vi "Close.vi"(8 "error in (no error)":errorcluster, 11 "Motions in":refnum<class "Motions.lvclass">) -> (0 "error out":errorcluster, 3 "Motions out":refnum<class "Motions.lvclass">)   [LabVIEW 2016, in "Hardware.lvlib" / "Motions.lvlib" / "Motions.lvclass"]
uses:
  <userlib>/Common Components/Hardware/Abstract System/Motions/Motions/Motions.lvclass
  <userlib>/Common Components/Hardware/Abstract System/Motions/Motions/Motions.lvclass/Motions.ctl
  <userlib>/Common Components/Hardware/Motor/Motor/Motor.lvclass
  <userlib>/Common Components/TriggerAction Q/TriggerAction Q/TriggerAction Q.lvclass
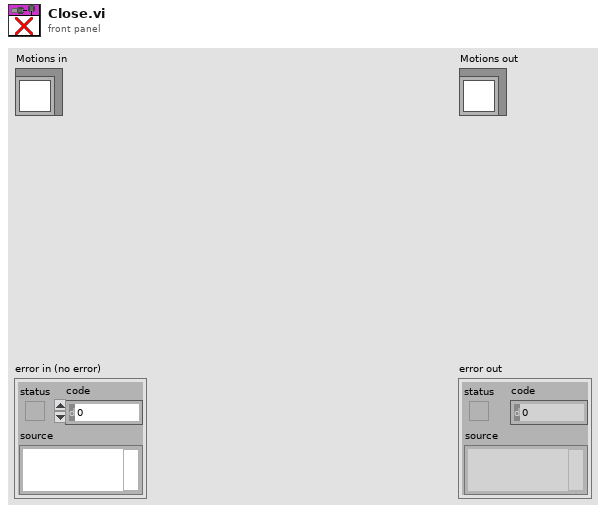
[diagram p1: front panel]
types:
  T1 = typedef "Hardware.lvlib/Motions.lvlib/Motions.lvclass/Motor States.ctl" = cluster{"Connected":bool, "Enabled":bool, "Moving Status":bool, "Soft Moving Status":bool, "Current Pos":dbl, "Target Pos":dbl, "Moving Dir (-1, 0, 1)":i32, "Error Status":bool, "Hard Limit+":bool, "Hard Limit-":bool, "Soft Limit+":bool, "Soft Limit-":bool, "History Dst Stack":refnum<queue>, "Motion Status":bool, "Motion TriggerAction Obj":refnum<class "TriggerAction Q.lvclass">}
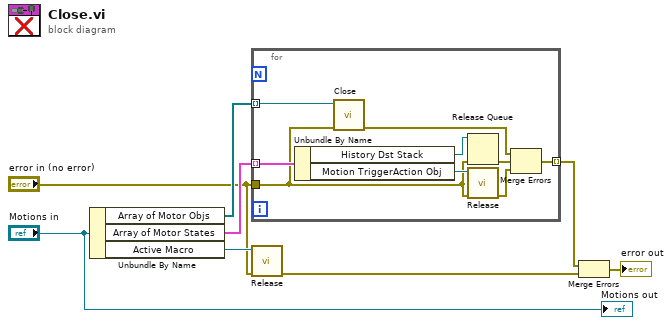
[diagram p0: block diagram]
diagram:
  n1 = Unbundle By Name("Motions in") -> ("Array of Motor Objs"=w7:refnum<class "Motor.lvclass">[], "Array of Motor States"=w4:T1[], "Active Macro"=w3:refnum<class "TriggerAction Q.lvclass">)
  n2 = for {
    tunnel: w7 -> [w17] mode=indexing
    tunnel: "error in (no error)" -> [w9]
    tunnel: [w12] -> w6 mode=indexing
    tunnel: w4 -> [w15] mode=indexing
    n3 = Unbundle By Name(w15) -> ("History Dst Stack"=w14:refnum<queue>, "Motion TriggerAction Obj"=w13:refnum<class "TriggerAction Q.lvclass">)
    n4 = call-dynamic "Close.vi"("error in (no error)"=w9, "CCD in"=w17) -> ("error out"=w16:errorcluster)  [unwired: 8 in, 1 out]
    n5 = Release Queue(queue=w14, error in (no error)=w9) -> (error out=w11:errorcluster)  [unwired: 1 in, 2 out]
    n6 = call <userlib>:"Release.vi"("error in (no error)"=w9, "TriggerAction in"=w13) -> ("error out"=w10:errorcluster)  [unwired: 8 in, 1 out]
    n7 = Merge Errors(w16, w11, w10) -> (w12:errorcluster)
  }
  n8 = call <userlib>:"Release.vi"("error in (no error)"="error in (no error)", "TriggerAction in"=w3) -> ("error out"=w1:errorcluster)  [unwired: 8 in, 1 out]
  n9 = Merge Errors(w6, w1) -> (→"error out":errorcluster)
  "Motions out" <- "Motions in"
